vi "CONEX_FG.vi"() -> ()   [LabVIEW 2010]
uses:
  <vilib>/Instr/_visa.llb/VISA Open Access Mode.ctl
  <vilib>/Instr/_visa.llb/VISA Configure Serial Port (Instr).vi
panel:
  out "concatenated string":string
  out "String 2":string
  in  "read":bool
  in  "stop":bool
  in  "send":bool
  in  "String":string
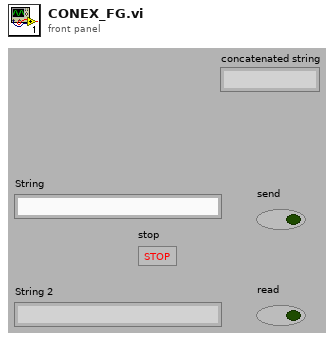
[diagram p1: front panel]
types:
  T1 = typedef "VISA Open Access Mode.ctl" = u32
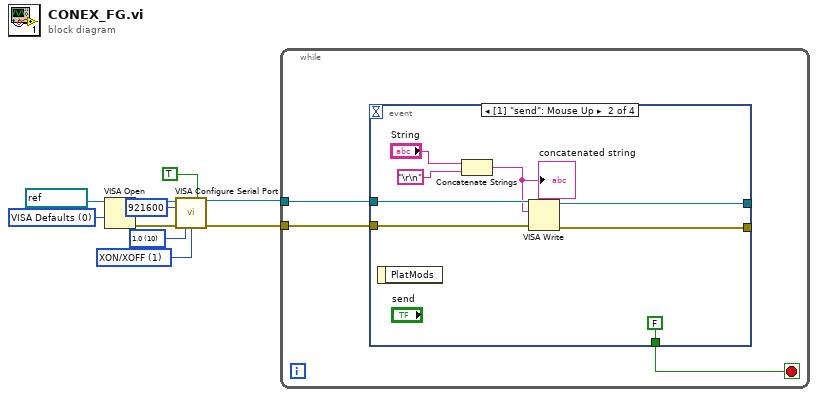
[diagram p0: block diagram]
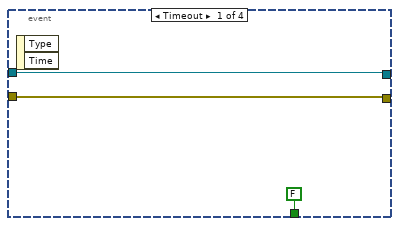
[diagram p2: hidden frame]
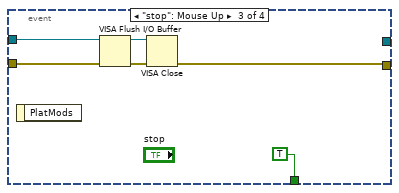
[diagram p3: hidden frame]
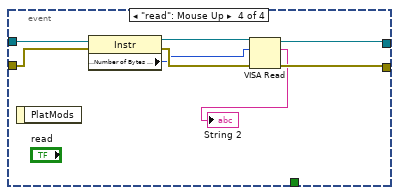
[diagram p4: hidden frame]
diagram:
  w2 = u16 1 items=["None", "XON/XOFF", "RTS/CTS", "XON/XOFF & RTS/CTS", "DTR/DSR", "XON/XOFF & DTR/DSR"] ("flow control (0:none)")
  w3 = u16 10 items=["1.0"=10, "1.5"=15, "2.0"=20] ("stop bits (10: 1 bit)")
  w9 = T1 0 items=["VISA Defaults"=0, "Exclusive Lock"=1, "Load Configured Settings"=4] ("Access Mode")
  n1 = VISA Open(access mode=w9, VISA resource name=refnum<visa-resource-name> "COM3") -> (VISA resource name=w8:refnum<visa-resource-name>, error out=w7:errorcluster)  [unwired: 3 in]
  n2 = call-poly "VISA Configure Serial Port"("VISA resource name"=w8, "Enable Termination\nChar (T)"=TRUE ("Enable Termination\nChar (T)"), "baud rate (9600)"=u32 921600, "error in (no error)"=w7, "stop bits (10: 1 bit)"=w3, "flow control (0:none)"=w2) -> ("VISA resource name out"=w6:refnum<visa-resource-name>, "error out"=w5:errorcluster)  [unwired: 8 in]
  n3 = while {
    tunnel: w6 -> [w13]
    tunnel: w5 -> [w12]
    stop <- w11 stop-if-true
    n4 = event shown="[1] \"send\": Mouse Up" {
      selector: _ -> [_ _ _ _]
      dyn-events: _ -> [_ _ _ _]
      timeout: _ -> [_ _ _ _]
      tunnel: w13 -> [w16 w24 w27 w38]
      tunnel: w12 -> [w15 w23 w26 w37]
      tunnel: [w16 w22 _ w33] -> _
      tunnel: [w15 w21 w25 w32] -> _
      tunnel: [FALSE FALSE TRUE _] -> w11
      event Timeout {
        n5 = event-data() -> ()  [unwired: 1 in, 2 out]
      }
      event "send": Mouse Up {
        n6 = event-data() -> ()  [unwired: 1 in, 1 out]
        n7 = Concatenate Strings("String", "\r\n") -> (w17:string)
        "concatenated string" <- w17
        n8 = VISA Write(VISA resource name=w24, write buffer=w17, error in (no error)=w23) -> (VISA resource name out=w22:refnum<visa-resource-name>, error out=w21:errorcluster)  [unwired: 1 out]
      }
      event "stop": Mouse Up {
        n9 = event-data() -> ()  [unwired: 1 in, 1 out]
        n10 = VISA Flush I/O Buffer(VISA resource name=w27, error in (no error)=w26) -> (VISA resource name out=w28:refnum<visa-resource-name>, error out=w29:errorcluster)  [unwired: 1 in]
        n11 = VISA Close(VISA resource name=w28, error in (no error)=w29) -> (error out=w25:errorcluster)
      }
      event "read": Mouse Up {
        n12 = event-data() -> ()  [unwired: 1 in, 1 out]
        n13 = property class="Instr"(reference=w38, error in=w37) -> (reference out=w36:refnum<visa-resource-name>, error out=w35:errorcluster, "Serial Settings:Number of Bytes at Serial Port"=w34:u32)
        n14 = VISA Read(VISA resource name=w36, byte count=w34, error in (no error)=w35) -> (VISA resource name out=w33:refnum<visa-resource-name>, read buffer=→"String 2":string, error out=w32:errorcluster)  [unwired: 1 out]
      }
    }
  }
